vi "DAQ.vi"() -> ()   [LabVIEW 2018]
panel:
  in  "stop":bool
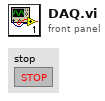
[diagram p1: front panel]
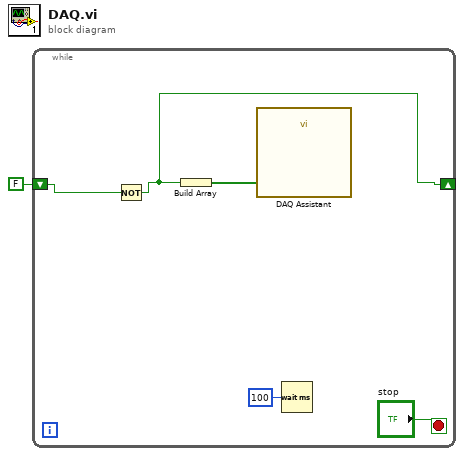
[diagram p0: block diagram]
diagram:
  n1 = while {
    shift-right: [w3] -> _
    shift-left: FALSE -> [w2]
    stop <- "stop" stop-if-true
    n2 = Not(x=w2) -> (.not. x?=w3:bool)
    n3 = Build Array(w3) -> (w4:bool[])
    n4 = call "DAQ Assistant"("data"=w4) -> ()  [unwired: 17 in, 2 out]
    n5 = Wait (ms)(milliseconds to wait=u32 100) -> ()  [unwired: 1 out]
  }
